vi "InitVIEW.vi"(8 "error in (no error)":errorcluster, 10 "VIEW":refnum<class "VIEW.lvclass">, 11 "CONTROLLER in":refnum<class "CONTROLLER.lvclass">) -> (0 "error out":errorcluster, 3 "CONTROLLER out":refnum<class "CONTROLLER.lvclass">)   [LabVIEW 2013, in "CONTROLLER.lvclass"]
uses:
  CONTROLLER.lvclass
  View/base/VIEW.lvclass
  CONTROLLER.lvclass/CONTROLLER.ctl
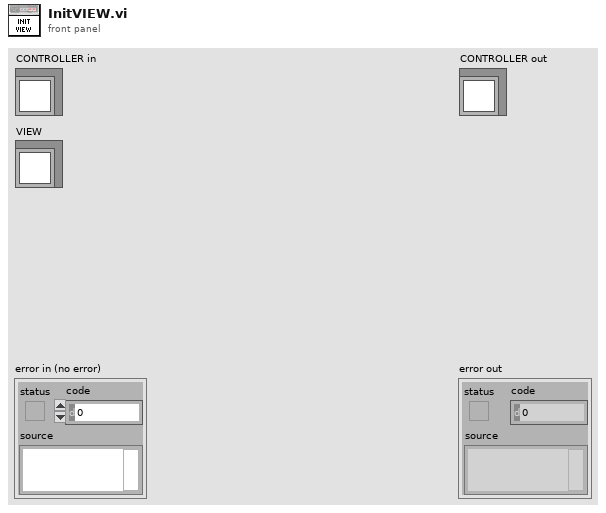
[diagram p1: front panel]
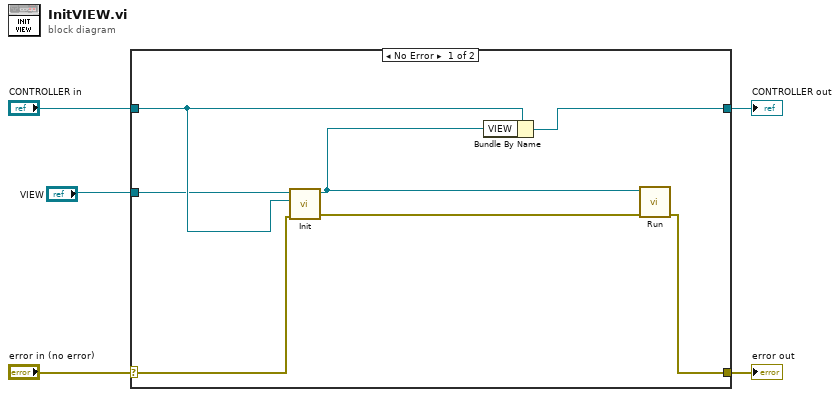
[diagram p0: block diagram]
diagram:
  n1 = case shown="No Error" "error in (no error)" {
    selector: "error in (no error)" -> [w8 w14]
    tunnel: [w7 w14] -> w4
    tunnel: [w12 w13] -> w2
    tunnel: "CONTROLLER in" -> [w11 w13]
    tunnel: "VIEW" -> [w6 _]
    frame No Error {
      n2 = call-dynamic "Init.vi"("error in (no error)"=w8, "CONTROLLER"=w11, "VIEW in"=w6) -> ("error out"=w9:errorcluster, "VIEW out"=w10:refnum<class "VIEW.lvclass">)  [unwired: 7 in]
      n3 = Bundle By Name(cluster=w11, "VIEW"=w10) -> (w12:refnum<class "CONTROLLER.lvclass">)
      n4 = call-dynamic "Run.vi"("error in (no error)"=w9, "VIEW in"=w10) -> ("error out"=w7:errorcluster)  [unwired: 8 in, 1 out]
    }
    frame Error {
    }
  }
  "error out" <- w4
  "CONTROLLER out" <- w2
